vi "classify error.vi"(8 "error to classify":errorcluster, 11 "TEC runtime in":refnum<class "TEC runtime.lvclass">) -> (0 "classified error":errorcluster, 2 "error classification":T1, 3 "TEC runtime out":refnum<class "TEC runtime.lvclass">)   [LabVIEW 2013, in "TEC runtime.lvclass"]
doc: "Allows a module to classify an error generated at any point during execution. This <b>error classification</b> can then be used by calling code to determine if execution can continue. In addition, this function can be used to allow a component to clear an error, convert an error to a warning, or attempt to recover from an error. Recovery may be attempted only if <b>attempt recovery?</b> is true."
uses:
  TEC runtime.lvclass
  <vilib>/NI/Tag Bus Module Framework/runtime/error classification.ctl
  <vilib>/NI/Tag Bus Module Framework/runtime/TBM module execution interface.lvclass
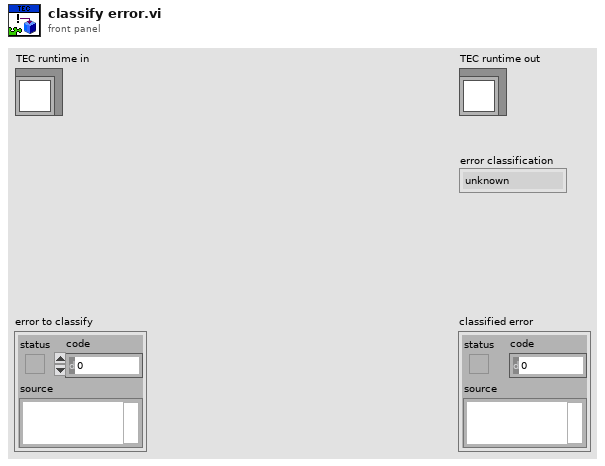
[diagram p1: front panel]
types:
  T1 = typedef "TBM module execution interface.lvclass/error classification.ctl" = enum16{"unknown", "none", "trivial", "recoverable", "critical"}
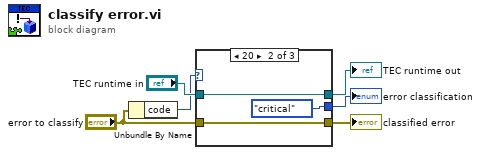
[diagram p0: block diagram]
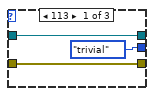
[diagram p2: hidden frame]
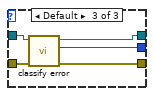
[diagram p3: hidden frame]
diagram:
  n1 = Unbundle By Name("error to classify") -> ("code"=w1:i32)
  n2 = case shown="20" w1 {
    tunnel: "error to classify" -> [w8 w11 w17]
    tunnel: [w8 w11 w16] -> w6
    tunnel: "TEC runtime in" -> [w9 w12 w15]
    tunnel: [w9 w12 w14] -> w4
    tunnel: [error_classification."trivial" ("error classification") error_classification."critical" ("error classification") w13] -> w3
    frame 113 {
    }
    frame 20 {
    }
    frame Default {
      n3 = call-parent "classify error.vi"("error to classify"=w17, "module in"=w15) -> ("classified error"=w16:errorcluster, "error classification"=w13:T1, "module out"=w14:refnum<class "TEC runtime.lvclass">)  [unwired: 7 in]
    }
  }
  "TEC runtime out" <- w4
  "error classification" <- w3
  "classified error" <- w6
